vi "Global display 4.vi"() -> ()   [LabVIEW 2017]
panel:
  in  "LAB deg C":T1
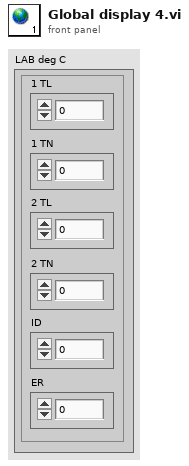
[diagram p1: front panel]
types:
  T1 = cluster{"1 TL":dbl, "1 TN":dbl, "2 TL":dbl, "2 TN":dbl, "ID":dbl, "ER":dbl}
diagram:
